vi "Variant to XY-Data.vi"(2 "error in (no error)":errorcluster, 3 "Value in":variant) -> (0 "error out":errorcluster, 1 "Value out":cluster{"X":dbl[], "Y":dbl[]}[](array[cluster]))   [LabVIEW 2019, in "graph_utilities.lvclass"]
uses:
  graph_utilities.lvclass
  <vilib>/Utility/Data Type/NI_Data Type.lvlib
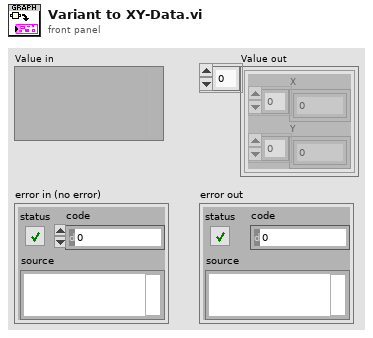
[diagram p1: front panel]
types:
  T1 = typedef "NI_Data Type.lvlib/Data Type.ctl" = enum8{"Invalid Type", "Void", "I8", "I16", "I32", "I64", "U8", "U16", "U32", "U64", "Single Float", "Double Float", "Extended Float", "Single Complex", "Double Complex", "Extended Complex", "Enum U8", "Enum U16", "Enum U32", "Enum U64", "Single Float With Unit", "Double Float With Unit", "Extended Float With Unit", "Single Complex with Unit", "Double Complex with Unit", "Extended Complex with Unit", "Boolean", "String", "Path", "Picture", "Tag", "Array", "Cluster", "Variant", "LV Variant", "Waveform", "Timestamp", "Digital Waveform", "Digital Data", "ExpressData", "Refnum", "External Data", "VI", "Poly VI", "LabVIEW Class Instance", "Fixed Point", "Set Collection", "Map Collection"}
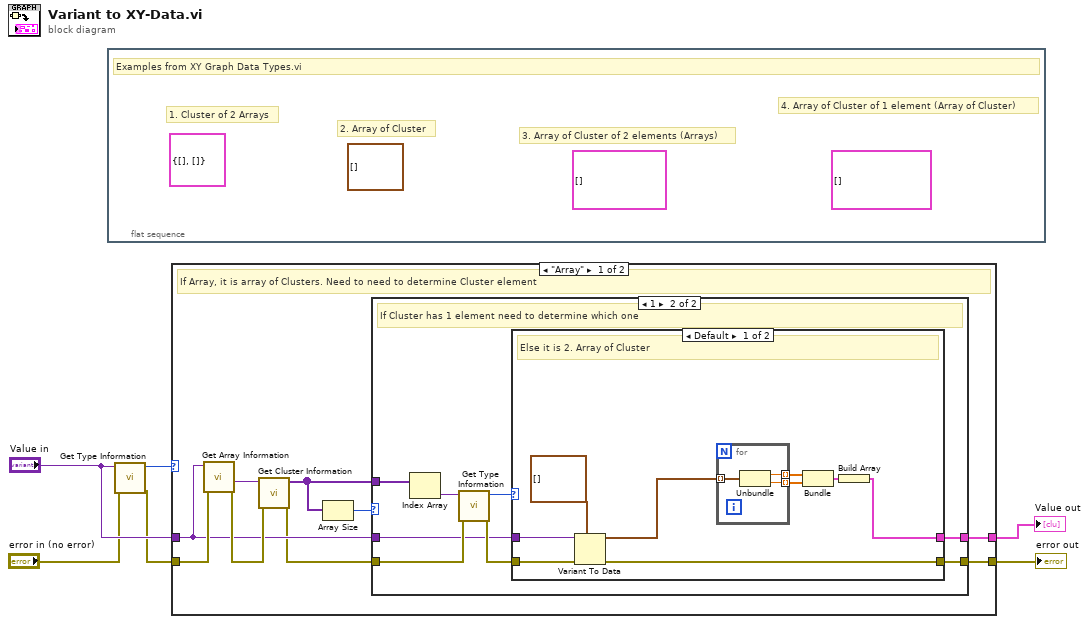
[diagram p0: block diagram]
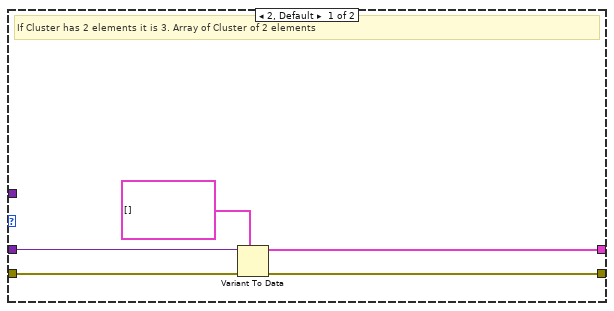
[diagram p2: hidden frame]
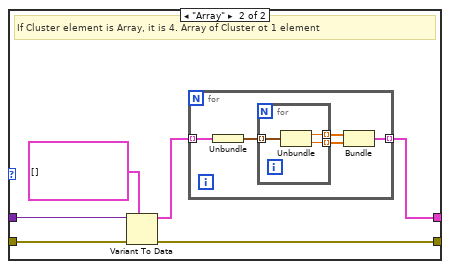
[diagram p3: hidden frame]
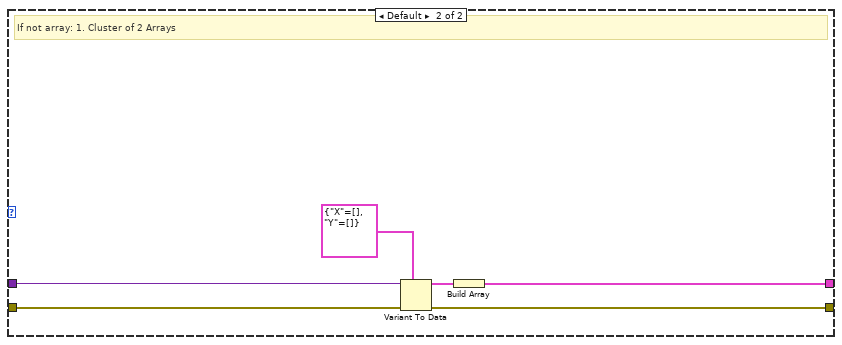
[diagram p4: hidden frame]
diagram:
  n1 = flat-sequence {
    frame #0 {
      (unwired) cluster{cluster{i32, dbl}[]}[] [] ("Multiple Plots (Array of X,Y Pairs)")
      (unwired) cluster{i32[], dbl[]}[] [] ("Multiple Plots (X Array and Y Array)")
      (unwired) cluster{i32[], dbl[]} {[], []} ("Single Plot (X Array and Y Array)")
      (unwired) cluster{i32, dbl}[] [] ("Single Plot (Array of X,Y Pairs)")
      # "4. Array of Cluster of 1 element (Array of Cluster)"
      # "3. Array of Cluster of 2 elements (Arrays)"
      # "2. Array of Cluster"
      # "1. Cluster of 2 Arrays"
      # "Examples from XY Graph Data Types.vi"
    }
  }
  n2 = call <vilib>:"Get Type Information.vi"("error in (no error)"="error in (no error)", "variant"="Value in") -> ("error out"=w2:errorcluster, "type"=w3:T1)  [unwired: 5 in, 3 out]
  n3 = case shown="\"Array\"" w3 {
    tunnel: [w10 w56] -> w6
    tunnel: [w12 w59] -> w5
    tunnel: w2 -> [w14 w58]
    tunnel: "Value in" -> [w11 w57]
    frame "Array" {
      # "If Array, it is array of Clusters. Need to need to determine Cluster element"
      n4 = call <vilib>:"Get Array Information.vi"("error in (no error)"=w14, "variant"=w11) -> ("error out"=w13:errorcluster, "array element data type"=w15:variant)  [unwired: 6 in, 2 out]
      n5 = call <vilib>:"Get Cluster Information.vi"("error in (no error)"=w13, "variant"=w15) -> ("error out"=w8:errorcluster, "cluster elements"=w7:variant[])  [unwired: 8 in]
      n6 = Array Size(array=w7) -> (size(s)=w9:i32)
      n7 = case shown="1" w9 {
        tunnel: w8 -> [w17 w26]
        tunnel: [w20 w25] -> w12
        tunnel: w11 -> [w16 w22]
        tunnel: [w18 w21] -> w10
        tunnel: w7 -> [_ w27]
        frame 2, Default {
          # "If Cluster has 2 elements it is 3. Array of Cluster of 2 elements"
          n8 = Variant To Data(error in=w17, type=cluster{"X":dbl[], "Y":dbl[]}[] [] ("XY Graph"), Variant=w16) -> (data=w18:cluster{"X":dbl[], "Y":dbl[]}[], error out=w20:errorcluster)
        }
        frame 1 {
          # "If Cluster has 1 element need to determine which one"
          n9 = Index Array(array=w27) -> (element=w28:variant)  [unwired: 1 in]
          n10 = call <vilib>:"Get Type Information.vi"("error in (no error)"=w26, "variant"=w28) -> ("error out"=w24:errorcluster, "type"=w23:T1)  [unwired: 5 in, 3 out]
          n11 = case shown="Default" w23 {
            tunnel: w24 -> [w37 w46]
            tunnel: [w30 w45] -> w25
            tunnel: w22 -> [w36 w44]
            tunnel: [w31 w41] -> w21
            frame Default {
              # "Else it is 2. Array of Cluster"
              n12 = Variant To Data(error in=w37, type=cluster{dbl, dbl}[] [] ("Single Plot (Array of X,Y Pairs)"), Variant=w36) -> (data=w29:cluster{dbl, dbl}[], error out=w30:errorcluster)
              n13 = for {
                tunnel: w29 -> [w40] mode=indexing
                tunnel: [w39] -> w34 mode=indexing
                tunnel: [w38] -> w33 mode=indexing
                n14 = Unbundle(w40) -> (w39:dbl, w38:dbl)
              }
              n15 = Bundle(w34, w33) -> (w32:cluster{dbl[], dbl[]})  [unwired: 1 in]
              n16 = Build Array(w32) -> (w31:cluster{dbl[], dbl[]}[])
            }
            frame "Array" {
              # "If Cluster element is Array, it is 4. Array of Cluster ot 1 element"
              n17 = Variant To Data(error in=w46, type=cluster{cluster{dbl, dbl}[]}[] [] ("Multiple Plots (Array of X,Y Pairs)"), Variant=w44) -> (data=w42:cluster{cluster{dbl, dbl}[]}[], error out=w45:errorcluster)
              n18 = for {
                tunnel: w42 -> [w51] mode=indexing
                tunnel: [w47] -> w41 mode=indexing
                n19 = Unbundle(w51) -> (w50:cluster{dbl, dbl}[])
                n20 = for {
                  tunnel: w50 -> [w54] mode=indexing
                  tunnel: [w53] -> w49 mode=indexing
                  tunnel: [w52] -> w48 mode=indexing
                  n21 = Unbundle(w54) -> (w53:dbl, w52:dbl)
                }
                n22 = Bundle(w49, w48) -> (w47:cluster{dbl[], dbl[]})  [unwired: 1 in]
              }
            }
          }
        }
      }
    }
    frame Default {
      # "If not array: 1. Cluster of 2 Arrays"
      n23 = Variant To Data(error in=w58, type=cluster{"X":dbl[], "Y":dbl[]} {"X"=[], "Y"=[]}, Variant=w57) -> (data=w60:cluster{"X":dbl[], "Y":dbl[]}, error out=w59:errorcluster)
      n24 = Build Array(w60) -> (w56:cluster{"X":dbl[], "Y":dbl[]}[])
    }
  }
  "Value out" <- w6
  "error out" <- w5
